vi "CCE MGLD PMJD PF SubVI011.vi"(1 "n20":dbl, 2 "n12":dbl, 3 "n02":dbl, 4 "n21":dbl, 5 "n03":dbl, 6 "n30":dbl, 7 "n11":dbl) -> (0 "Momentos Hu":T1)   [LabVIEW 2020]
doc: "Ceballos Conde Emanuel Meneses Gutiérrez Luis David Pineda Méndez Job Daniel 4MV6 Sistemas de visión artificial 2022/1 \nEste VI devuelve el arreglo de los momentos invariables Hu a partir de los parametros npq."
panel:
  # "Ceballos Conde Emanuel   -  Meneses Gutiérrez Luis David   -  Pineda Méndez Job Daniel 4MV6 Sistemas de visión artificial  2022/1             SubVI011"
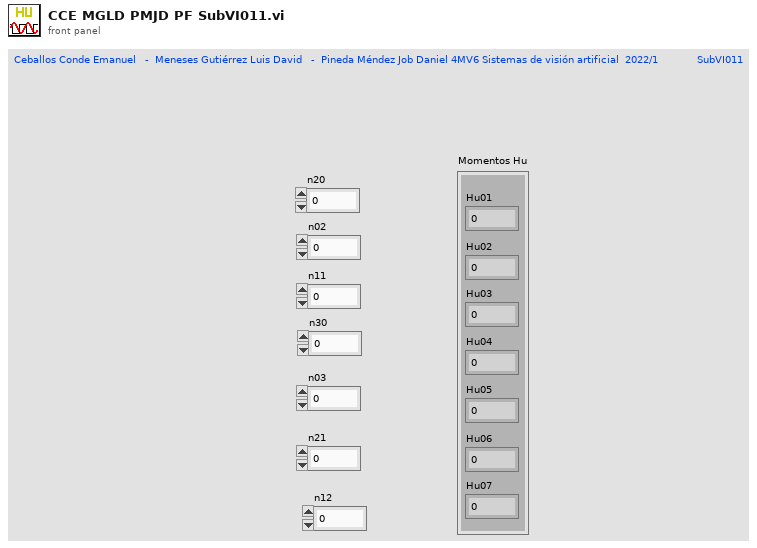
[diagram p1: front panel]
types:
  T1 = cluster{"Hu01":dbl, "Hu02":dbl, "Hu03":dbl, "Hu04":dbl, "Hu05":dbl, "Hu06":dbl, "Hu07":dbl}
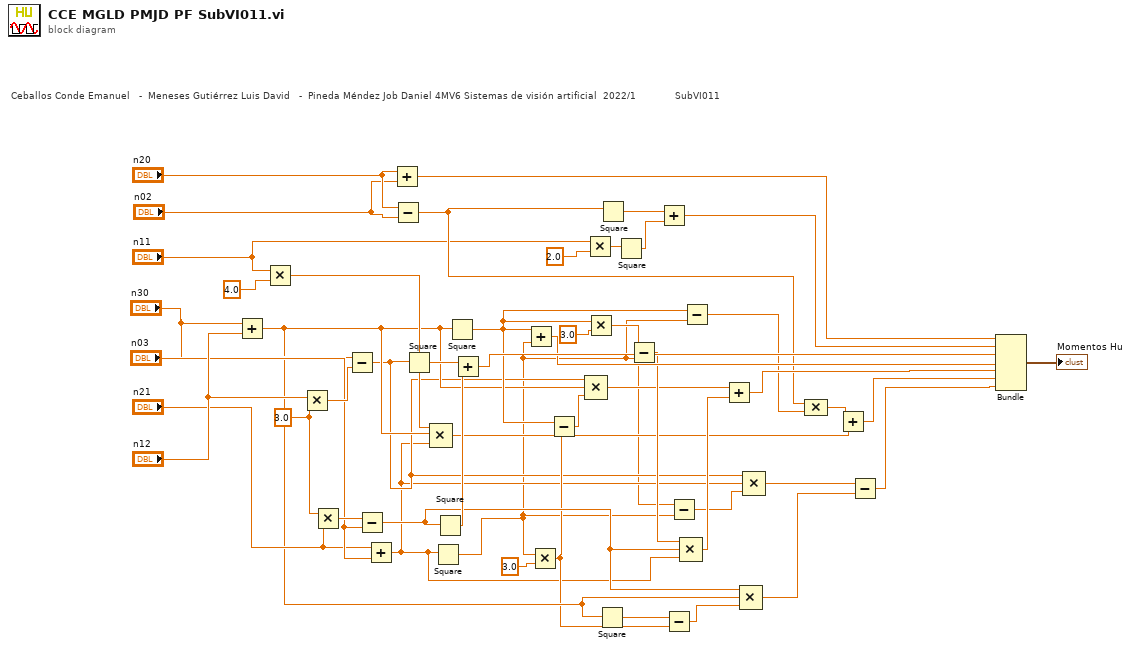
[diagram p0: block diagram]
diagram:
  w39 = 3.0 ("y")
  # "Ceballos Conde Emanuel   -  Meneses Gutiérrez Luis David   -  Pineda Méndez Job Daniel 4MV6 Sistemas de visión artificial  2022/1             SubVI011"
  n1 = Add(x="n30", y="n12") -> (x+y=w10:dbl)
  n2 = Multiply(x="n11", y=4.0) -> (x*y=w17:dbl)
  n3 = Multiply(x="n12", y=w39) -> (x*y=w41:dbl)
  n4 = Multiply(x=w39, y="n21") -> (x*y=w38:dbl)
  n5 = Subtract(x="n30", y=w41) -> (x-y=w7:dbl)
  n6 = Subtract(x=w38, y="n03") -> (x-y=w13:dbl)
  n7 = Add(x="n21", y="n03") -> (x+y=w6:dbl)
  n8 = Add(x="n20", y="n02") -> (x+y=w47:dbl)
  n9 = Subtract(x="n20", y="n02") -> (x-y=w23:dbl)
  n10 = Square(x=w7) -> (x^2=w40:dbl)
  n11 = Compound Arithmetic op=MULTIPLY(w17, w10, w6) -> (w16:dbl)
  n12 = Square(x=w6) -> (x^2=w3:dbl)
  n13 = Square(x=w13) -> (x^2=w37:dbl)
  n14 = Square(x=w10) -> (x^2=w21:dbl)
  n15 = Add(x=w40, y=w37) -> (x+y=w36:dbl)
  n16 = Add(x=w21, y=w3) -> (x+y=w32:dbl)
  n17 = Multiply(x=w3, y=3.0) -> (x*y=w9:dbl)
  n18 = Subtract(x=w21, y=w9) -> (x-y=w30:dbl)
  n19 = Multiply(x="n11", y=2.0) -> (x*y=w44:dbl)
  n20 = Compound Arithmetic op=MULTIPLY(w7, w10, w30) -> (w25:dbl)
  n21 = Multiply(x=w21, y=3.0) -> (x*y=w4:dbl)
  n22 = Square(x=w10) -> (x^2=w11:dbl)
  n23 = Square(x=w23) -> (x^2=w46:dbl)
  n24 = Square(x=w44) -> (x^2=w43:dbl)
  n25 = Subtract(x=w4, y=w3) -> (x-y=w27:dbl)
  n26 = Add(x=w46, y=w43) -> (x+y=w42:dbl)
  n27 = Subtract(x=w11, y=w9) -> (x-y=w12:dbl)
  n28 = Subtract(x=w4, y=w3) -> (x-y=w5:dbl)
  n29 = Compound Arithmetic op=MULTIPLY(w27, w13, w6) -> (w26:dbl)
  n30 = Subtract(x=w21, y=w3) -> (x-y=w22:dbl)
  n31 = Add(x=w25, y=w26) -> (x+y=w24:dbl)
  n32 = Compound Arithmetic op=MULTIPLY(w13, w10, w12) -> (w1:dbl)
  n33 = Compound Arithmetic op=MULTIPLY(w7, w6, w5) -> (w2:dbl)
  n34 = Compound Arithmetic op=MULTIPLY(w23, w22) -> (w20:dbl)
  n35 = Add(x=w20, y=w16) -> (x+y=w15:dbl)
  n36 = Subtract(x=w2, y=w1) -> (x-y=w8:dbl)
  n37 = Bundle(w47, w42, w36, w32, w24, w15, w8) -> (→"Momentos Hu":cluster{dbl, dbl, dbl, dbl, dbl, dbl, dbl})  [unwired: 1 in]
